vi "PCO_GetADCOperation.vi"(8 "error in (no error)":errorcluster {"code" format="%x"}, 11 "ph":u64) -> (0 "error out":errorcluster {"code" format="%x"}, 1 "wADCOperation":u16(ring) items=["", "single ADC", "dual ADC"], 2 "ErrorMessage":i32 format="%x", 3 "ph out":u64)   [LabVIEW 2019, in "SDK.lvlib" / "ImageSensor.lvlib"]
doc: "<b>Description:</b>\nThis function returns the ADC (analog / digital converter) operating mode (single / dual) currently used from the camera.\n\n<b>Supported camera type:</b>\nAll cameras\n\n<b>Descriptor dependency:</b>\nwNumADCsDESC"
uses:
  ImageSensor.lvlib
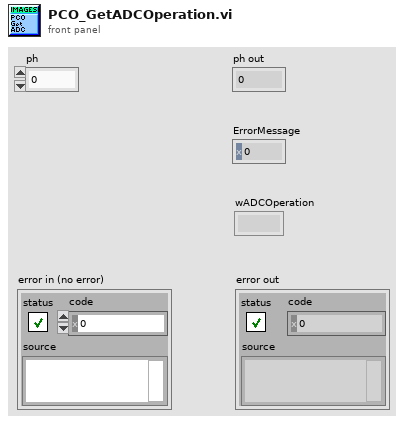
[diagram p1: front panel]
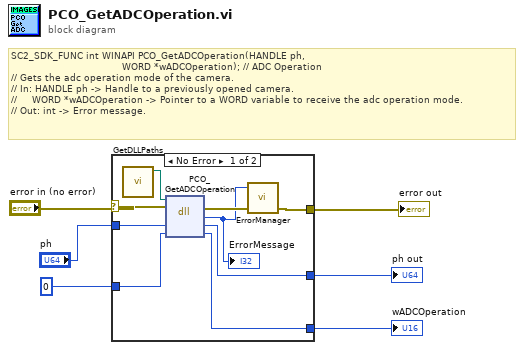
[diagram p0: block diagram]
diagram:
  # "SC2_SDK_FUNC int WINAPI PCO_GetADCOperation(HANDLE ph,\n                                     WORD *wADCOperation); // ADC Operation\n// Gets the adc operation mode of the camera.\n// In: HANDLE ph -> Handle to a previously opened camera.\n//     WORD *wADCOperation -> Pointer to a WORD variable to receive the adc operation mode.\n// Out: int -> Error message."
  n1 = case shown="No Error" "error in (no error)" {
    selector: "error in (no error)" -> [w11 w18]
    tunnel: "ph" -> [w15 w17]
    tunnel: [w14 w17] -> w5
    tunnel: u16 0 ("wADCOperation") -> [w13 w16]
    tunnel: [w12 w16] -> w3
    tunnel: [w10 w18] -> w2
    frame No Error {
      n2 = call "GetDLLPaths.vi"() -> ("SC2_Cam_Path"=w7:path)  [unwired: 9 in, 2 out]
      n3 = dll-call lib="?" fn="PCO_GetADCOperation"(path in=w7, error in=w11, "ph"=w15, "wADCOperation"=w13) -> (error out=w9:errorcluster, "return type"=w8:i32, "ph"=w14:u64, "wADCOperation"=w12:u16)  [unwired: 1 in, 1 out]
      "ErrorMessage" <- w8
      n4 = call "ErrorManager.vi"("error in (no error)"=w9, "error code"=w8) -> ("error out"=w10:errorcluster)  [unwired: 3 in]
    }
    frame Error {
    }
  }
  "ph out" <- w5
  "wADCOperation" <- w3
  "error out" <- w2
